vi "log analysis_gps.vi"() -> ()   [LabVIEW 2019] (continued)
\n\t\n15:46:26.6\tlog_raw\tgps_raw\t#INSPVAXA,USB3,0,50.5,FINESTEERING,2107,283604.650,02000000,471d,15824;INS_ALIGNMENT_COMPLETE,INS_RTKFIXED,37.37126199805,126.72219243143,7.9649,22.3000,0.0555,0.0695,0.0079,0.560896506,-1.435960650,267.028457385,0.4379,0.2961,0.5759,0.1131,0.0925,0.0784,0.0963,0.1009,5.1528,0f000001,0*81aa449e\n\tsystem status\tnormal 2 27.900000 0 0\trobot status\t120.229744\t125.611680\t7.964900\t0.560897\t-1.435961\t-177.028457\t-0.015000\t0.004000\n\t\n15:46:27.1\tlog_raw\tgps_raw\t\tsystem status\tnormal 2 27.900000 0 0\trobot status\t120.247613\t125.622386\t7.963000\t0.540052\t-1.322126\t-177.100128\t0.000000\t0.000000\n\t\n15:46:27.6\tlog_raw\tgps_raw\t\tsystem status\tnormal 2 27.900000 0 0\trobot status\t120.240000\t125.629099\t7.960700\t0.528374\t-1.345188\t-177.091097\t-0.003000\t0.005000\n\t\n15:46:28.1\tlog_raw\tgps_raw\t\tsystem status\tnormal 2 27.900000 0 0\trobot status\t120.240346\t125.635985\t7.958800\t0.528065\t-1.344161\t-177.088301\t0.000000\t0.000000\n\t\n15:46:28.6\tlog_raw\tgps_raw\t\tsystem status\tnormal 2 27.900000 0 0\trobot status\t120.241214\t125.638419\t7.957500\t0.527317\t-1.343603\t-177.097018\t0.000000\t0.000000\n\t\n15:46:29.1\tlog_raw\tgps_raw\t#INSPVAXA,USB3,0,45.0,FINESTEERING,2107,283607.150,02000000,471d,15824;INS_ALIGNMENT_COMPLETE,INS_RTKFIXED,37.37126226214,126.72219256337,7.9563,22.3000,0.0507,-0.0122,0.0067,0.527133772,-1.343948140,267.105174531,0.4402,0.2962,0.5756,0.1140,0.0925,0.0784,0.0963,0.1009,5.1518,0f000001,0*37532215\n\tsystem status\tnormal 2 27.900000 0 0\trobot status\t120.241431\t125.640990\t7.956300\t0.527134\t-1.343948\t-177.105175\t0.000000\t0.000000\n\t\n15:46:29.6\tlog_raw\tgps_raw\t#INSPVAXA,USB3,0,45.0,FINESTEERING,2107,283607.650,02000000,471d,15824;INS_ALIGNMENT_COMPLETE,INS_RTKFIXED,37.37126225847,126.72219257288,7.9545,22.3000,0.0487,-0.0117,0.0063,0.526769970,-1.341614130,267.120484585,0.4402,0.2962,0.5756,0.1140,0.0925,0.0784,0.0963,0.1009,5.1518,0f000001,0*097e3cbc\n\tsystem status\tnormal 2 27.900000 0 0\trobot status\t120.242273\t125.640582\t7.954500\t0.526770\t-1.341614\t-177.120485\t0.000000\t0.000000\n\t\n15:46:30.1\tlog_raw\tgps_raw\t\tsystem status\tnormal 2 27.900000 0 0\trobot status\t120.242654\t125.640475\t7.952800\t0.525450\t-1.341849\t-177.138025\t0.000000\t0.000000\n\t\n15:46:30.6\tlog_raw\tgps_raw\t\tsystem status\tnormal 2 27.900000 0 0\trobot status\t120.243154\t125.638122\t7.950900\t0.525220\t-1.343908\t-177.155087\t0.000000\t0.000000\n\t\n15:46:31.1\tlog_raw\tgps_raw\t\tsystem status\tnormal 2 27.900000 0 0\trobot status\t120.243352\t125.636540\t7.949400\t0.526035\t-1.344537\t-177.171645\t0.000000\t0.000000\n\t\n15:46:31.6\tlog_raw\tgps_raw\t\tsystem status\tnormal 2 27.900000 0 0\trobot status\t120.243773\t125.634214\t7.948000\t0.525760\t-1.343630\t-177.189591\t0.000000\t0.000000\n\t\n15:46:32.1\tlog_raw\tgps_raw\t\tsystem status\tnormal 2 27.900000 0 0\trobot status\t120.244034\t125.632347\t7.946800\t0.526232\t-1.341058\t-177.213820\t0.031000\t0.016000\n\t\n15:46:32.6\tlog_raw\tgps_raw\t\tsystem status\tnormal 2 27.800000 0 0\trobot status\t120.157560\t125.623590\t7.944400\t0.518356\t-1.205486\t-177.172033\t0.334000\t0.069000\n\t\n15:46:33.1\tlog_raw\tgps_raw\t\tsystem status\tnormal 2 27.900000 0 0\trobot status\t119.992825\t125.615194\t7.941000\t0.761003\t-1.235075\t-177.213040\t0.247000\t0.083000\n\t\n15:46:33.6\tlog_raw\tgps_raw\t\tsystem status\tnormal 2 27.800000 0 0\trobot status\t119.859694\t125.608416\t7.939500\t0.865415\t-0.962854\t-177.206885\t0.328000\t0.009000\n\t\n15:46:34.1\tlog_raw\tgps_raw\t\tsystem status\tnormal 2 27.900000 0 0\trobot status\t119.720756\t125.602946\t7.937700\t0.944420\t-0.675187\t-177.209566\t0.305000\t-0.006000\n\t\n15:46:34.6\tlog_raw\tgps_raw\t\tsystem status\tnormal 2 27.900000 0 0\trobot status\t119.607706\t125.601145\t7.935300\t1.235838\t-0.694517\t-176.982274\t0.053000\t0.017000\n\t\n15:46:35.2\tlog_raw\tgps_raw\t\tsystem status\tnormal 2 27.900000 0 0\trobot status\t119.498199\t125.596969\t7.933300\t1.155764\t-0.364011\t-177.058938\t0.315000\t0.047000\n\t\n15:46:35.7\tlog_raw\tgps_raw\t\tsystem status\tnormal 2 27.800000 0 0\trobot status\t119.370674\t125.593736\t7.932700\t1.037480\t-0.074198\t-176.883392\t0.323000\t0.000000\n\t\n15:46:36.2\tlog_raw\tgps_raw\t\tsystem status\tnormal 2 27.800000 0 0\trobot status\t119.227990\t125.592351\t7.933400\t1.079023\t0.069605\t-176.833003\t0.331000\t-0.050000\n\t\n15:46:36.7\tlog_raw\tgps_raw\t\tsystem status\tnormal 2 27.900000 0 0\trobot status\t119.087343\t125.592838\t7.934300\t1.129008\t0.093647\t-176.796316\t0.344000\t-0.082000\n\t\n15:46:37.2\tlog_raw\tgps_raw\t\tsystem status\tnormal 2 27.900000 0 0\trobot status\t118.945543\t125.594297\t7.935700\t1.235778\t0.057060\t-176.780369\t0.373000\t-0.127000\n\t\n15:46:37.7\tlog_raw\tgps_raw\t\tsystem status\tnormal 2 27.900000 0 0\trobot status\t118.803696\t125.594493\t7.937600\t1.216235\t-0.108384\t-176.748954\t0.357000\t-0.086000\n\t\n15:46:38.2\tlog_raw\tgps_raw\t\tsystem status\tnormal 2 27.800000 0 0\trobot status\t118.664225\t125.596035\t7.939400\t1.263594\t-0.402279\t-176.659906\t0.284000\t0.032000\n\t\n15:46:38.7\tlog_raw\tgps_raw\t\tsystem status\tnormal 2 27.900000 0 0\trobot status\t118.524850\t125.597283\t7.939600\t1.404144\t-0.659021\t-176.624250\t0.281000\t0.019000\n\t\n15:46:39.2\tlog_raw\tgps_raw\t\tsystem status\tnormal 2 27.900000 0 0\trobot status\t118.381157\t125.599793\t7.940000\t1.598406\t-0.888086\t-176.601260\t0.360000\t-0.098000\n\t\n15:46:39.7\tlog_raw\tgps_raw\t\tsystem status\tnormal 2 27.800000 0 0\trobot status\t118.277291\t125.603881\t7.941400\t1.566580\t-0.870870\t-176.521281\t0.316000\t0.024000\n\t\n15:46:40.2\tlog_raw\tgps_raw\t\tsystem status\tnormal 2 27.900000 0 0\trobot status\t118.128647\t125.607002\t7.942100\t1.627827\t-0.936186\t-176.519460\t0.217000\t0.054000\n\t\n15:46:40.7\tlog_raw\tgps_raw\t\tsystem status\tnormal 2 27.900000 0 0\trobot status\t117.982836\t125.609853\t7.941800\t1.720683\t-0.789013\t-176.481119\t0.260000\t0.048000\n\t\n15:46:41.2\tlog_raw\tgps_raw\t\tsystem status\tnormal 2 27.900000 0 0\trobot status\t117.844520\t125.613894\t7.942800\t1.697089\t-0.531895\t-176.383127\t0.285000\t0.052000\n\t\n15:46:41.7\tlog_raw\tgps_raw\t#INSPVAXA,USB3,0,49.5,FINESTEERING,2107,283619.700,02000000,471d,15824;INS_ALIGNMENT_COMPLETE,INS_RTKFIXED,37.37126206039,126.72216378783,7.9456,22.3000,0.0422,-0.2948,0.0158,1.718323220,-0.193748450,266.266037782,0.4350,0.2957,0.5763,0.1125,0.0925,0.0784,0.0965,0.1009,5.1330,0f000001,0*8635b490\n\tsystem status\tnormal 2 27.800000 0 0\trobot status\t117.692541\t125.618635\t7.945600\t1.718323\t-0.193748\t-176.266038\t0.383000\t-0.099000\n\t\n15:46:42.2\tlog_raw\tgps_raw\t\tsystem status\tnormal 2 27.800000 0 0\trobot status\t117.566611\t125.621702\t7.946700\t1.591710\t-0.089350\t-176.226869\t0.365000\t-0.094000\n\t\n15:46:42.7\tlog_raw\tgps_raw\t\tsystem status\tnormal 2 27.800000 0 0\trobot status\t117.417289\t125.623343\t7.946200\t1.490039\t-0.163044\t-176.175266\t0.376000\t-0.104000\n\t\n15:46:43.2\tlog_raw\tgps_raw\t\tsystem status\tnormal 2 27.800000 0 0\trobot status\t117.272242\t125.625795\t7.946400\t1.307058\t-0.220578\t-176.105754\t0.263000\t0.075000\n\t\n15:46:43.7\tlog_raw\tgps_raw\t\tsystem status\tnormal 2 27.800000 0 0\trobot status\t117.130621\t125.627578\t7.947200\t1.149741\t-0.274212\t-175.977532\t0.361000\t-0.089000\n\t\n15:46:44.2\tlog_raw\tgps_raw\t#INSPVAXA,USB3,0,47.5,FINESTEERING,2107,283622.200,02000000,471d,15824;INS_ALIGNMENT_COMPLETE,INS_RTKFIXED,37.37126217486,126.72215605148,7.9488,22.3000,0.0265,-0.2568,0.0016,0.953197769,-0.264991418,265.735651965,0.4362,0.2956,0.5763,0.1134,0.0927,0.0784,0.0965,0.1010,5.1347,0f000001,0*d1c7aea0\n\tsystem status\tnormal 2 27.800000 0 0\trobot status\t117.007267\t125.631349\t7.948800\t0.953198\t-0.264991\t-175.735652\t0.219000\t0.009000\n\t\n15:46:44.7\tlog_raw\tgps_raw\t\tsystem status\tnormal 2 27.800000 0 0\trobot status\t116.858071\t125.629441\t7.947800\t0.820028\t-0.582510\t-175.730144\t0.220000\t0.076000\n\t\n15:46:45.2\tlog_raw\tgps_raw\t#INSPVAXA,USB3,0,49.5,FINESTEERING,2107,283623.200,02000000,471d,15824;INS_ALIGNMENT_COMPLETE,INS_RTKFIXED,37.37126215352,126.72215258792,7.9480,22.3000,0.0351,-0.2613,0.0231,0.659350525,-0.553290360,265.516937653,0.4377,0.2954,0.5765,0.1123,0.0931,0.0784,0.0965,0.1010,5.1353,0f000001,0*f37e3ed0\n\tsystem status\tnormal 2 27.800000 0 0\trobot status\t116.700471\t125.628985\t7.948000\t0.659351\t-0.553290\t-175.516938\t0.236000\t0.095000\n\t\n15:46:45.7\tlog_raw\tgps_raw\t\tsystem status\tnormal 2 27.800000 0 0\trobot status\t116.570534\t125.627968\t7.947400\t0.491368\t-0.548221\t-175.479442\t0.356000\t-0.073000\n\t\n15:46:46.2\tlog_raw\tgps_raw\t\tsystem status\tnormal 2 27.800000 0 0\trobot status\t116.422797\t125.627372\t7.946500\t0.429298\t-0.761102\t-175.343158\t0.340000\t-0.050000\n\t\n15:46:46.7\tlog_raw\tgps_raw\t\tsystem status\tnormal 2 27.800000 0 0\trobot status\t116.278573\t125.625026\t7.945600\t0.327130\t-0.869350\t-175.264091\t0.333000\t-0.039000\n\t\n15:46:47.2\tlog_raw\tgps_raw\t#INSPVAXA,USB3,0,49.5,FINESTEERING,2107,283625.200,02000000,471d,15824;INS_ALIGNMENT_COMPLETE,INS_RTKFIXED,37.37126210638,126.72214606046,7.9447,22.3000,0.0217,-0.2754,0.0073,0.236515804,-0.792213520,265.180407825,0.4366,0.2950,0.5766,0.1123,0.0931,0.0784,0.0964,0.1010,5.1329,0f000001,0*acc95a4e\n\tsystem status\tnormal 2 27.800000 0 0\trobot status\t116.122279\t125.623761\t7.944700\t0.236516\t-0.792214\t-175.180408\t0.347000\t-0.074000\n\t\n15:46:47.7\tlog_raw\tgps_raw\t#INSPVAXA,USB3,0,49.5,FINESTEERING,2107,283625.700,02000000,471d,15824;INS_ALIGNMENT_COMPLETE,INS_RTKFIXED,37.37126208247,126.72214443464,7.9445,22.3000,0.0140,-0.2813,0.0048,0.046048670,-0.588797871,265.114785763,0.4366,0.2950,0.5766,0.1123,0.0931,0.0784,0.0964,0.1010,5.1329,0f000001,0*ce0a2a96\n\tsystem status\tnormal 2 27.800000 0 0\trobot status\t115.978267\t125.621109\t7.944500\t0.046049\t-0.588798\t-175.114786\t0.250000\t0.075000\n\t\n15:46:48.2\tlog_raw\tgps_raw\t#INSPVAXA,USB3,0,48.0,FINESTEERING,2107,283626.200,02000000,471d,15824;INS_ALIGNMENT_COMPLETE,INS_RTKFIXED,37.37126206372,126.72214280060,7.9445,22.3000,0.0212,-0.2855,0.0048,-0.004156486,-0.311026110,265.065225665,0.4366,0.2949,0.5766,0.1123,0.0931,0.0784,0.0963,0.1010,5.1300,0f000001,0*7442e942\n\tsystem status\tnormal 2 27.900000 0 0\trobot status\t115.833526\t125.619030\t7.944500\t-0.004156\t-0.311026\t-175.065226\t0.377000\t-0.106000\n\t\n15:46:48.7\tlog_raw\tgps_raw\t\tsystem status\tnormal 2 27.800000 0 0\trobot status\t115.708474\t125.615805\t7.943800\t-0.132371\t0.068230\t-174.996675\t0.252000\t0.082000\n\t\n15:46:49.2\tlog_raw\tgps_raw\t#INSPVAXA,USB3,0,48.5,FINESTEERING,2107,283627.200,02000000,471d,15824;INS_ALIGNMENT_COMPLETE,INS_RTKFIXED,37.37126201142,126.72213963218,7.9431,22.3000,0.0278,-0.2914,0.0131,-0.197757356,0.430555181,264.900646420,0.4366,0.2949,0.5768,0.1127,0.0931,0.0784,0.0962,0.1009,5.1266,0f000001,0*c875f714\n\tsystem status\tnormal 2 27.800000 0 0\trobot status\t115.552873\t125.613230\t7.943100\t-0.197757\t0.430555\t-174.900646\t0.372000\t-0.099000\n\t\n15:46:49.7\tlog_raw\tgps_raw\t\tsystem status\tnormal 2 27.800000 0 0\trobot status\t115.421996\t125.610470\t7.941400\t-0.273360\t0.391133\t-174.920780\t0.299000\t0.008000\n\t\n15:46:50.2\tlog_raw\tgps_raw\t\tsystem status\tnormal 2 27.900000 0 0\trobot status\t115.278884\t125.608053\t7.940600\t-0.346212\t0.271634\t-174.916641\t0.299000\t0.000000\n\t\n15:46:50.7\tlog_raw\tgps_raw\t#INSPVAXA,USB3,0,48.0,FINESTEERING,2107,283628.700,02000000,471d,15824;INS_ALIGNMENT_COMPLETE,INS_RTKFIXED,37.37126191178,126.72213473323,7.9380,22.3000,0.0177,-0.2797,-0.0032,-0.623534384,0.011887408,264.986854356,0.4375,0.2949,0.5768,0.1127,0.0930,0.0784,0.0962,0.1009,5.1221,0f000001,0*2b23c567\n\tsystem status\tnormal 2 27.900000 0 0\trobot status\t115.118932\t125.602177\t7.938000\t-0.623534\t0.011887\t-174.986854\t0.294000\t0.000000\n\t\n15:46:51.2\tlog_raw\tgps_raw\t#INSPVAXA,USB3,0,44.0,FINESTEERING,2107,283629.200,02000000,471d,15824;INS_ALIGNMENT_COMPLETE,INS_RTKFIXED,37.37126187751,126.72213308389,7.9364,22.3000,0.0207,-0.2899,-0.0036,-0.719101472,-0.426401600,265.021502859,0.4380,0.2949,0.5768,0.1123,0.0930,0.0784,0.0961,0.1009,5.1171,0f000001,0*92ebbc5f\n\tsystem status\tnormal 2 27.900000 0 0\trobot status\t114.972836\t125.598376\t7.936400\t-0.719101\t-0.426402\t-175.021503\t0.296000\t0.002000\n\t\n15:46:51.7\tlog_raw\tgps_raw\t#INSPVAXA,USB3,0,44.0,FINESTEERING,2107,283629.700,02000000,471d,15824;INS_ALIGNMENT_COMPLETE,INS_RTKFIXED,37.37126184367,126.72213142920,7.9356,22.3000,0.0231,-0.2981,-0.0100,-0.725013495,-0.732992105,265.121442983,0.4380,0.2949,0.5768,0.1123,0.0930,0.0784,0.0961,0.1009,5.1171,0f000001,0*6a5775b3\n\tsystem status\tnormal 2 27.900000 0 0\trobot status\t114.826266\t125.594622\t7.935600\t-0.725013\t-0.732992\t-175.121443\t0.302000\t0.000000\n\t\n15:46:52.2\tlog_raw\tgps_raw\t#INSPVAXA,USB3,0,47.0,FINESTEERING,2107,283630.200,02000000,471d,15824;INS_ALIGNMENT_COMPLETE,INS_RTKFIXED,37.37126181957,126.72212981940,7.9352,22.3000,0.0233,-0.2888,-0.0019,-0.675781239,-0.810566304,265.160131093,0.4376,0.2949,0.5768,0.1123,0.0928,0.0784,0.0961,0.1009,5.1128,0f000001,0*27ca04ea\n\tsystem status\tnormal 2 27.900000 0 0\trobot status\t114.683673\t125.591949\t7.935200\t-0.675781\t-0.810566\t-175.160131\t0.296000\t0.005000\n\t\n15:46:52.7\tlog_raw\tgps_raw\t#INSPVAXA,USB3,0,47.0,FINESTEERING,2107,283630.700,02000000,471d,15824;INS_ALIGNMENT_COMPLETE,INS_RTKFIXED,37.37126178591,126.72212819473,7.9347,22.3000,0.0150,-0.2861,-0.0012,-0.714770911,-0.869266848,265.221494891,0.4376,0.2949,0.5768,0.1123,0.0928,0.0784,0.0961,0.1009,5.1128,0f000001,0*aed2de40\n\tsystem status\tnormal 2 27.900000 0 0\trobot status\t114.539762\t125.588216\t7.934700\t-0.714771\t-0.869267\t-175.221495\t0.298000\t0.001000\n\t\n15:46:53.2\tlog_raw\tgps_raw\t#INSPVAXA,USB3,0,42.0,FINESTEERING,2107,283631.200,02000000,471d,15824;INS_ALIGNMENT_COMPLETE,INS_RTKFIXED,37.37126175832,126.72212651988,7.9323,22.3000,0.0193,-0.2829,-0.0000,-0.656726245,-0.814467356,265.316189024,0.4372,0.2950,0.5769,0.1123,0.0926,0.0784,0.0961,0.1009,5.1101,0f000001,0*d1b6c699\n\tsystem status\tnormal 2 27.900000 0 0\trobot status\t114.391407\t125.585156\t7.932300\t-0.656726\t-0.814467\t-175.316189\t0.295000\t-0.016000\n\t\n15:46:53.7\tlog_raw\tgps_raw\t#INSPVAXA,USB3,0,42.0,FINESTEERING,2107,283631.700,02000000,471d,15824;INS_ALIGNMENT_COMPLETE,INS_RTKFIXED,37.37126176860,126.72212533305,7.9296,22.3000,0.0361,-0.3378,-0.0103,-0.428138119,-0.668837581,265.144757660,0.4372,0.2950,0.5769,0.1123,0.0926,0.0784,0.0961,0.1009,5.1101,0f000001,0*53a99c66\n\tsystem status\tnormal 2 27.900000 0 0\trobot status\t114.286279\t125.586298\t7.929600\t-0.428138\t-0.668838\t-175.144758\t0.298000\t-0.003000\n\t\n15:46:54.2\tlog_raw\tgps_raw\t\tsystem status\tnormal 2 27.900000 0 0\trobot status\t114.123517\t125.583422\t7.925900\t-0.165245\t-0.957147\t-175.287983\t0.290000\t0.016000\n\t\n15:46:54.7\tlog_raw\tgps_raw\t#INSPVAXA,USB3,0,48.5,FINESTEERING,2107,283632.700,02000000,471d,15824;INS_ALIGNMENT_COMPLETE,INS_RTKFIXED,37.37126172516,126.72212196595,7.9217,22.3000,0.0261,-0.3154,-0.0017,-0.080275609,-1.010698207,265.307907457,0.4366,0.2951,0.5768,0.1127,0.0925,0.0784,0.0961,0.1008,5.1091,0f000001,0*c955826f\n\tsystem status\tnormal 2 27.900000 0 0\trobot status\t113.988027\t125.581481\t7.921700\t-0.080276\t-1.010698\t-175.307907\t0.298000\t-0.007000\n\t\n15:46:55.2\tlog_raw\tgps_raw\t#INSPVAXA,USB3,0,44.5,FINESTEERING,2107,283633.200,02000000,471d,15824;INS_ALIGNMENT_COMPLETE,INS_RTKFIXED,37.37126169079,126.72212014716,7.9199,22.3000,0.0199,-0.3002,0.0131,-0.062381377,-1.283391784,265.467989015,0.4356,0.2952,0.5768,0.1125,0.0925,0.0784,0.0961,0.1008,5.1096,0f000001,0*29ba6107\n\tsystem status\tnormal 2 27.900000 0 0\trobot status\t113.826921\t125.577668\t7.919900\t-0.062381\t-1.283392\t-175.467989\t0.302000\t-0.007000\n\t\n15:46:55.7\tlog_raw\tgps_raw\t#INSPVAXA,USB3,0,44.5,FINESTEERING,2107,283633.700,02000000,471d,15824;INS_ALIGNMENT_COMPLETE,INS_RTKFIXED,37.37126167129,126.72211861960,7.9201,22.3000,0.0266,-0.3162,-0.0026,-0.118708398,-1.041509272,265.462110158,0.4356,0.2952,0.5768,0.1125,0.0925,0.0784,0.0961,0.1008,5.1096,0f000001,0*f2130a3a\n\tsystem status\tnormal 2 27.900000 0 0\trobot status\t113.691613\t125.575506\t7.920100\t-0.118708\t-1.041509\t-175.462110\t0.303000\t0.002000\n\t\n15:46:56.2\tlog_raw\tgps_raw\t#INSPVAXA,USB3,0,50.5,FINESTEERING,2107,283634.200,02000000,471d,15824;INS_ALIGNMENT_COMPLETE,INS_RTKFIXED,37.37126166951,126.72211687193,7.9193,22.3000,0.0345,-0.2873,0.0162,0.231523125,-0.963780299,265.599746817,0.4352,0.2955,0.5769,0.1123,0.0929,0.0784,0.0961,0.1009,5.1105,0f000001,0*34468b3e\n\tsystem status\tnormal 2 27.900000 0 0\trobot status\t113.536807\t125.575311\t7.919300\t0.231523\t-0.963780\t-175.599747\t0.296000\t-0.010000\n\t\n15:46:56.7\tlog_raw\tgps_raw\t#INSPVAXA,USB3,0,50.5,FINESTEERING,2107,283634.700,02000000,471d,15824;INS_ALIGNMENT_COMPLETE,INS_RTKFIXED,37.37126165383,126.72211529605,7.9180,22.3000,0.0293,-0.3222,-0.0026,0.312038300,-0.626564523,265.688696868,0.4352,0.2955,0.5769,0.1123,0.0929,0.0784,0.0961,0.1009,5.1105,0f000001,0*7451a5d1\n\tsystem status\tnormal 2 27.900000 0 0\trobot status\t113.397218\t125.573572\t7.918000\t0.312038\t-0.626565\t-175.688697\t0.309000\t-0.004000\n\t\n15:46:57.2\tlog_raw\tgps_raw\t#INSPVAXA,USB3,0,48.5,FINESTEERING,2107,283635.200,02000000,471d,15824;INS_ALIGNMENT_COMPLETE,INS_RTKFIXED,37.37126163429,126.72211368866,7.9175,22.3000,0.0223,-0.3021,-0.0082,0.186097207,-0.250317479,265.804263291,0.4352,0.2960,0.5769,0.1124,0.0928,0.0784,0.0961,0.1009,5.1109,0f000001,0*57ac3a22\n\tsystem status\tnormal 2 27.900000 0 0\trobot status\t113.254838\t125.571406\t7.917500\t0.186097\t-0.250317\t-175.804263\t0.298000\t-0.006000\n\t\n15:46:57.7\tlog_raw\tgps_raw\t#INSPVAXA,USB3,0,48.5,FINESTEERING,2107,283635.700,02000000,471d,15824;INS_ALIGNMENT_COMPLETE,INS_RTKFIXED,37.37126159822,126.72211206599,7.9179,22.3000,0.0256,-0.3005,0.0044,-0.110995339,-0.087789516,265.935244450,0.4352,0.2960,0.5769,0.1124,0.0928,0.0784,0.0961,0.1009,5.1109,0f000001,0*fb1bd604\n\tsystem status\tnormal 2 27.900000 0 0\trobot status\t113.111105\t125.567404\t7.917900\t-0.110995\t-0.087790\t-175.935244\t0.296000\t-0.006000\n\t\n15:46:58.2\tlog_raw\tgps_raw\t\tsystem status\tnormal 2 27.900000 0 0\trobot status\t112.986609\t125.566337\t7.918000\t-0.168558\t-0.306352\t-176.034603\t0.281000\t0.003000\n\t\n15:46:58.7\tlog_raw\tgps_raw\t#INSPVAXA,USB3,0,43.0,FINESTEERING,2107,283636.700,02000000,471d,15824;INS_ALIGNMENT_COMPLETE,INS_RTKFIXED,37.37126158491,126.72210906167,7.9172,22.3000,0.0261,-0.3515,0.0074,-0.153804874,-0.423258614,266.149623913,0.4359,0.2963,0.5769,0.1124,0.0927,0.0784,0.0961,0.1009,5.1114,0f000001,0*20701ae8\n\tsystem status\tnormal 2 27.900000 0 0\trobot status\t112.844987\t125.565931\t7.917200\t-0.153805\t-0.423259\t-176.149624\t0.318000\t-0.009000\n\t\n15:46:59.2\tlog_raw\tgps_raw\t#INSPVAXA,USB3,0,48.5,FINESTEERING,2107,283637.200,02000000,471d,15824;INS_ALIGNMENT_COMPLETE,INS_RTKFIXED,37.37126157389,126.72210741579,7.9182,22.3000,0.0244,-0.2694,0.0184,-0.300056136,-0.600225307,266.307903185,0.4364,0.2964,0.5768,0.1122,0.0926,0.0784,0.0961,0.1009,5.1119,0f000001,0*6c5dc01c\n\tsystem status\tnormal 2 27.900000 0 0\trobot status\t112.699198\t125.564710\t7.918200\t-0.300056\t-0.600225\t-176.307903\t0.277000\t-0.009000\n\t\n15:46:59.7\tlog_raw\tgps_raw\t#INSPVAXA,USB3,0,48.5,FINESTEERING,2107,283637.700,02000000,471d,15824;INS_ALIGNMENT_COMPLETE,INS_RTKFIXED,37.37126156174,126.72210572455,7.9205,22.3000,0.0137,-0.2979,0.0107,-0.519565417,-0.746251495,266.511093088,0.4364,0.2964,0.5768,0.1122,0.0926,0.0784,0.0961,0.1009,5.1119,0f000001,0*d93f2085\n\tsystem status\tnormal 2 27.900000 0 0\trobot status\t112.549390\t125.563363\t7.920500\t-0.519565\t-0.746251\t-176.511093\t0.294000\t-0.009000\n\t\n15:47:00.2\tlog_raw\tgps_raw\t#INSPVAXA,USB3,0,51.0,FINESTEERING,2107,283638.200,02000000,471d,15824;INS_ALIGNMENT_COMPLETE,INS_RTKFIXED,37.37126155440,126.72210403454,7.9211,22.3000,0.0270,-0.3337,0.0126,-0.860556856,-0.781571793,266.718697356,0.4367,0.2965,0.5770,0.1123,0.0925,0.0784,0.0961,0.1009,5.1124,0f000001,0*3b4b6ae8\n\tsystem status\tnormal 2 27.900000 0 0\trobot status\t112.399692\t125.562551\t7.921100\t-0.860557\t-0.781572\t-176.718697\t0.302000\t-0.016000\n\t\n15:47:00.7\tlog_raw\tgps_raw\t#INSPVAXA,USB3,0,51.0,FINESTEERING,2107,283638.700,02000000,471d,15824;INS_ALIGNMENT_COMPLETE,INS_RTKFIXED,37.37126156669,126.72210242363,7.9200,22.3000,0.0334,-0.3133,0.0178,-0.896958447,-0.619411990,266.906112882,0.4367,0.2965,0.5770,0.1123,0.0925,0.0784,0.0961,0.1009,5.1124,0f000001,0*cef03a1f\n\tsystem status\tnormal 2 27.900000 0 0\trobot status\t112.257000\t125.563916\t7.920000\t-0.896958\t-0.619412\t-176.906113\t0.296000\t-0.004000\n\t\n15:47:01.2\tlog_raw\tgps_raw\t#INSPVAXA,USB3,0,50.0,FINESTEERING,2107,283639.200,02000000,471d,15824;INS_ALIGNMENT_COMPLETE,INS_RTKFIXED,37.37126157899,126.72210075579,7.9190,22.3000,0.0338,-0.2994,0.0184,-0.981388962,-0.616865309,267.067890648,0.4364,0.2961,0.5771,0.1123,0.0925,0.0784,0.0961,0.1009,5.1135,0f000001,0*21baf340\n\tsystem status\tnormal 2 27.900000 0 0\trobot status\t112.109266\t125.565284\t7.919000\t-0.981389\t-0.616865\t-177.067891\t0.292000\t0.000000\n\t\n15:47:01.7\tlog_raw\tgps_raw\t#INSPVAXA,USB3,0,50.0,FINESTEERING,2107,283639.700,02000000,471d,15824;INS_ALIGNMENT_COMPLETE,INS_RTKFIXED,37.37126158948,126.72209911436,7.9198,22.3000,0.0295,-0.3287,0.0146,-1.013704154,-0.682043166,267.265330343,0.4364,0.2961,0.5771,0.1123,0.0925,0.0784,0.0961,0.1009,5.1135,0f000001,0*ee73127b\n\tsystem status\tnormal 2 27.900000 0 0\trobot status\t111.963871\t125.566450\t7.919800\t-1.013704\t-0.682043\t-177.265330\t0.302000\t-0.009000\n\t\n15:47:02.2\tlog_raw\tgps_raw\t#INSPVAXA,USB3,0,49.5,FINESTEERING,2107,283640.200,02000000,471d,15824;INS_ALIGNMENT_COMPLETE,INS_RTKFIXED,37.37126161750,126.72209746371,7.9213,22.3000,0.0430,-0.3344,0.0134,-0.961284284,-0.929903840,267.457563863,0.4362,0.2958,0.5770,0.1123,0.0925,0.0784,0.0961,0.1009,5.1150,0f000001,0*e2e7a72b\n\tsystem status\tnormal 2 27.900000 0 0\trobot status\t111.817659\t125.569561\t7.921300\t-0.961284\t-0.929904\t-177.457564\t0.305000\t-0.007000\n\t\n15:47:02.7\tlog_raw\tgps_raw\t#INSPVAXA,USB3,0,49.5,FINESTEERING,2107,283640.700,02000000,471d,15824;INS_ALIGNMENT_COMPLETE,INS_RTKFIXED,37.37126164969,126.72209583664,7.9226,22.3000,0.0427,-0.3200,0.0053,-1.010366927,-1.135102181,267.635350069,0.4362,0.2958,0.5770,0.1123,0.0925,0.0784,0.0961,0.1009,5.1150,0f000001,0*6b674dca\n\tsystem status\tnormal 2 27.900000 0 0\trobot status\t111.673535\t125.573136\t7.922600\t-1.010367\t-1.135102\t-177.635350\t0.299000\t-0.002000\n\t\n15:47:03.2\tlog_raw\tgps_raw\t#DUALANTENNAHEADINGA,USB3,0,50.0,FINESTEERING,2107,283641.200,02000000,d426,15824;INSUFFICIENT_OBS,NONE,-1.000000000,0.000000000,0.000000000,0.0,0.000000000,0.000000000,\"631T\",11,4,4,3,04,00,20,02*472a6cda\n\tsystem status\tnormal 2 27.900000 0 0\trobot status\t111.525039\t125.579051\t7.923500\t-0.873522\t-1.303089\t-177.784444\t0.296000\t0.000000\n\t\n15:47:03.7\tlog_raw\tgps_raw\t#INSPVAXA,USB3,0,50.0,FINESTEERING,2107,283641.700,02000000,471d,15824;INS_ALIGNMENT_COMPLETE,INS_RTKFIXED,37.37126176584,126.72209246619,7.9228,22.3000,0.0335,-0.3477,0.0031,-0.698463635,-1.495934209,267.964863954,0.4360,0.2957,0.5769,0.1125,0.0925,0.0784,0.0961,0.1009,5.1165,0f000001,0*ca9d9e5e\n\tsystem status\tnormal 2 27.900000 0 0\trobot status\t111.374987\t125.586031\t7.922800\t-0.698464\t-1.495934\t-177.964864\t0.302000\t0.004000\n\t\n15:47:04.2\tlog_raw\tgps_raw\t#INSPVAXA,USB3,0,50.0,FINESTEERING,2107,283642.200,02000000,471d,15824;INS_ALIGNMENT_COMPLETE,INS_RTKFIXED,37.37126183344,126.72209071714,7.9215,22.3000,0.0370,-0.3263,0.0036,-0.535216936,-1.667310153,268.031771555,0.4354,0.2957,0.5768,0.1127,0.0926,0.0784,0.0961,0.1009,5.1177,0f000001,0*11bec665\n\tsystem status\tnormal 2 27.900000 0 0\trobot status\t111.220059\t125.593535\t7.921500\t-0.535217\t-1.667310\t-178.031772\t0.300000\t-0.003000\n\t\n15:47:04.7\tlog_raw\tgps_raw\t#DUALANTENNAHEADINGA,USB3,0,50.0,FINESTEERING,2107,283642.700,02000000,d426,15824;INSUFFICIENT_OBS,NONE,-1.000000000,0.000000000,0.000000000,0.0,0.000000000,0.000000000,\"631T\",12,4,4,3,04,00,20,03*f200c6d7\n\tsystem status\tnormal 2 27.900000 0 0\trobot status\t111.081969\t125.600643\t7.920400\t-0.422501\t-1.714756\t-178.135075\t0.296000\t0.006000\n\t\n15:47:05.2\tlog_raw\tgps_raw\t#DUALANTENNAHEADINGA,USB3,0,50.5,FINESTEERING,2107,283643.200,02000000,d426,15824;INSUFFICIENT_OBS,NONE,-1.000000000,0.000000000,0.000000000,0.0,0.000000000,0.000000000,\"631T\",14,4,4,3,04,00,20,02*f76a0e1e\n\tsystem status\tnormal 2 27.900000 0 0\trobot status\t110.939369\t125.607555\t7.918700\t-0.466356\t-1.548228\t-178.190993\t0.304000\t0.001000\n\t\n15:47:05.7\tlog_raw\tgps_raw\t#INSPVAXA,USB3,0,50.5,FINESTEERING,2107,283643.700,02000000,471d,15824;INS_ALIGNMENT_COMPLETE,INS_RTKFIXED,37.37126202513,126.72208597859,7.9183,22.3000,0.0299,-0.3163,0.0088,-0.418582783,-1.196326458,268.184941514,0.4349,0.2958,0.5767,0.1124,0.0926,0.0784,0.0961,0.1010,5.1181,0f000001,0*962e1d48\n\tsystem status\tnormal 2 27.900000 0 0\trobot status\t110.800326\t125.614816\t7.918300\t-0.418583\t-1.196326\t-178.184942\t0.297000\t0.006000\n\t\n15:47:06.2\tlog_raw\tgps_raw\t#INSPVAXA,USB3,0,50.0,FINESTEERING,2107,283644.200,02000000,471d,15824;INS_ALIGNMENT_COMPLETE,INS_RTKFIXED,37.37126209425,126.72208434200,7.9172,22.3000,0.0360,-0.2950,0.0056,-0.334802719,-0.884110622,268.233385323,0.4347,0.2959,0.5767,0.1122,0.0926,0.0784,0.0961,0.1010,5.1180,0f000001,0*78a9edf8\n\tsystem status\tnormal 2 27.900000 0 0\trobot status\t110.655359\t125.622489\t7.917200\t-0.334803\t-0.884111\t-178.233385\t0.299000\t-0.001000\n\t\n15:47:06.7\tlog_raw\tgps_raw\t#INSPVAXA,USB3,0,50.0,FINESTEERING,2107,283644.700,02000000,471d,15824;INS_ALIGNMENT_COMPLETE,INS_RTKFIXED,37.37126215178,126.72208275426,7.9159,22.3000,0.0303,-0.2952,0.0021,-0.296302250,-0.633495852,268.293666475,0.4347,0.2959,0.5767,0.1122,0.0926,0.0784,0.0961,0.1010,5.1180,0f000001,0*8db6baa1\n\tsystem status\tnormal 2 27.900000 0 0\trobot status\t110.514720\t125.628876\t7.915900\t-0.296302\t-0.633496\t-178.293666\t0.298000\t-0.001000\n\t\n15:47:07.2\tlog_raw\tgps_raw\t#INSPVAXA,USB3,0,46.0,FINESTEERING,2107,283645.200,02000000,471d,15824;INS_ALIGNMENT_COMPLETE,INS_RTKFIXED,37.37126220166,126.72208110110,7.9146,22.3000,0.0357,-0.3070,0.0007,-0.345507272,-0.608999756,268.311610368,0.4352,0.2960,0.5768,0.1123,0.0926,0.0784,0.0961,0.1011,5.1185,0f000001,0*f711e95a\n\tsystem status\tnormal 2 27.900000 0 0\trobot status\t110.368285\t125.634414\t7.914600\t-0.345507\t-0.609000\t-178.311610\t0.287000\t0.026000\n\t\n15:47:07.7\tlog_raw\tgps_raw\t#DUALANTENNAHEADINGA,USB3,0,46.0,FINESTEERING,2107,283645.700,02000000,d426,15824;INSUFFICIENT_OBS,NONE,-1.000000000,0.000000000,0.000000000,0.0,0.000000000,0.000000000,\"631T\",14,4,4,3,04,00,20,03*e6910734\n\tsystem status\tnormal 2 27.900000 0 0\trobot status\t110.227517\t125.638786\t7.914100\t-0.511260\t-0.771457\t-178.296151\t0.302000\t0.015000\n\t\n15:47:08.2\tlog_raw\tgps_raw\t#INSPVAXA,USB3,0,45.5,FINESTEERING,2107,283646.200,02000000,471d,15824;INS_ALIGNMENT_COMPLETE,INS_RTKFIXED,37.37126228996,126.72207792557,7.9145,22.3000,0.0424,-0.3064,0.0070,-0.583777876,-0.970443227,268.202528664,0.4357,0.2960,0.5768,0.1124,0.0925,0.0784,0.0961,0.1011,5.1194,0f000001,0*211ff137\n\tsystem status\tnormal 2 27.900000 0 0\trobot status\t110.087002\t125.644217\t7.914500\t-0.583778\t-0.970443\t-178.202529\t0.286000\t0.027000\n\t\n15:47:08.7\tlog_raw\tgps_raw\t#INSPVAXA,USB3,0,45.5,FINESTEERING,2107,283646.700,02000000,471d,15824;INS_ALIGNMENT_COMPLETE,INS_RTKFIXED,37.37126233833,126.72207631349,7.9144,22.3000,0.0451,-0.2992,0.0137,-0.600671632,-1.104685881,268.101292386,0.4357,0.2960,0.5768,0.1124,0.0925,0.0784,0.0961,0.1011,5.1194,0f000001,0*24418ec0\n\tsystem status\tnormal 2 27.900000 0 0\trobot status\t109.944207\t125.649587\t7.914400\t-0.600672\t-1.104686\t-178.101292\t0.253000\t0.080000\n\t\n15:47:09.2\tlog_raw\tgps_raw\t#DUALANTENNAHEADINGA,USB3,0,48.5,FINESTEERING,2107,283647.200,02000000,d426,15824;INSUFFICIENT_OBS,NONE,-1.000000000,0.000000000,0.000000000,0.0,0.000000000,0.000000000,\"631T\",13,4,4,3,04,00,20,03*e3593a63\n\tsystem status\tnormal 2 27.800000 0 0\trobot status\t109.798996\t125.654285\t7.915100\t-0.711305\t-1.244972\t-178.007017\t0.294000\t0.028000\n\t\n15:47:09.7\tlog_raw\tgps_raw\t#INSPVAXA,USB3,0,48.5,FINESTEERING,2107,283647.700,02000000,471d,15824;INS_ALIGNMENT_COMPLETE,INS_RTKFIXED,37.37126242655,126.72207309668,7.9156,22.3000,0.0394,-0.3060,0.0118,-0.639679760,-1.236455959,267.822984990,0.4363,0.2960,0.5769,0.1123,0.0925,0.0784,0.0961,0.1011,5.1206,0f000001,0*6bb51677\n\tsystem status\tnormal 2 27.800000 0 0\trobot status\t109.659267\t125.659382\t7.915600\t-0.639680\t-1.236456\t-177.822985\t0.313000\t-0.004000\n\t\n15:47:10.2\tlog_raw\tgps_raw\t#INSPVAXA,USB3,0,48.0,FINESTEERING,2107,283648.200,02008000,471d,15824;INS_ALIGNMENT_COMPLETE,INS_RTKFIXED,37.37126246801,126.72207154325,7.9155,22.3000,0.0354,-0.2935,0.0108,-0.510675062,-1.137543161,267.571098751,0.4364,0.2959,0.5770,0.1124,0.0925,0.0784,0.0961,0.1011,5.1221,0f000001,0*c4dadb2f\n\tsystem status\tnormal 2 27.800000 0 0\trobot status\t109.521667\t125.663985\t7.915500\t-0.510675\t-1.137543\t-177.571099\t0.406000\t-0.159000\n\t\n15:47:10.7\tlog_raw\tgps_raw\t#INSPVAXA,USB3,0,48.0,FINESTEERING,2107,283648.700,02008000,471d,15824;INS_ALIGNMENT_COMPLETE,INS_RTKFIXED,37.37126248707,126.72206994787,7.9152,22.3000,0.0198,-0.2907,0.0205,-0.532213630,-1.121566976,267.351964744,0.4364,0.2959,0.5770,0.1124,0.0925,0.0784,0.0961,0.1011,5.1221,0f000001,0*5feed5da\n\tsystem status\tnormal 2 27.800000 0 0\trobot status\t109.380351\t125.666103\t7.915200\t-0.532214\t-1.121567\t-177.351965\t0.257000\t0.071000\n\t\n15:47:11.2\tlog_raw\tgps_raw\t#INSPVAXA,USB3,0,50.5,FINESTEERING,2107,283649.200,02008000,471d,15824;INS_ALIGNMENT_COMPLETE,INS_RTKFIXED,37.37126248971,126.72206839810,7.9149,22.3000,0.0089,-0.2933,0.0096,-0.659725734,-0.970229399,267.160180872,0.4369,0.2958,0.5772,0.1125,0.0925,0.0784,0.0961,0.1011,5.1235,0f000001,0*081a7c85\n\tsystem status\tnormal 2 27.800000 0 0\trobot status\t109.243075\t125.666397\t7.914900\t-0.659726\t-0.970229\t-177.160181\t0.269000\t0.067000\n\t\n15:47:11.7\tlog_raw\tgps_raw\t#INSPVAXA,USB3,0,50.5,FINESTEERING,2107,283649.700,02008000,471d,15824;INS_ALIGNMENT_COMPLETE,INS_RTKFIXED,37.37126248182,126.72206686817,7.9130,22.3000,0.0195,-0.2818,0.0147,-0.676677557,-0.877493738,266.924781860,0.4369,0.2958,0.5772,0.1125,0.0925,0.0784,0.0961,0.1011,5.1235,0f000001,0*7b64dc48\n\tsystem status\tnormal 2 27.800000 0 0\trobot status\t109.107556\t125.665523\t7.913000\t-0.676678\t-0.877494\t-176.924782\t0.304000\t0.005000\n\t\n15:47:12.2\tlog_raw\tgps_raw\t#INSPVAXA,USB3,0,51.0,FINESTEERING,2107,283650.200,02008000,471d,15824;INS_ALIGNMENT_COMPLETE,INS_RTKFIXED,37.37126249199,126.72206547845,7.9115,22.3000,0.0164,-0.3260,0.0139,-0.484645802,-0.829453687,266.635151565,0.4374,0.2957,0.5772,0.1135,0.0925,0.0784,0.0961,0.1011,5.1243,0f000001,0*b0320f40\n\tsystem status\tnormal 2 27.800000 0 0\trobot status\t108.984457\t125.666654\t7.911500\t-0.484646\t-0.829454\t-176.635152\t0.250000\t0.091000\n\t\n15:47:12.7\tlog_raw\tgps_raw\t#INSPVAXA,USB3,0,51.0,FINESTEERING,2107,283650.700,02008000,471d,15824;INS_ALIGNMENT_COMPLETE,INS_RTKFIXED,37.37126248591,126.72206385137,7.9107,22.3000,0.0102,-0.2983,0.0161,-0.427862387,-0.984462668,266.224829667,0.4374,0.2957,0.5772,0.1135,0.0925,0.0784,0.0961,0.1011,5.1243,0f000001,0*ccab10f5\n\tsystem status\tnormal 2 27.800000 0 0\trobot status\t108.840333\t125.665981\t7.910700\t-0.427862\t-0.984463\t-176.224830\t0.318000\t-0.010000\n\t\n15:47:13.2\tlog_raw\tgps_raw\t#INSPVAXA,USB3,0,46.5,FINESTEERING,2107,283651.200,02008000,471d,15824;INS_ALIGNMENT_COMPLETE,INS_RTKFIXED,37.37126247297,126.72206225341,7.9105,22.3000,-0.0025,-0.2931,0.0133,-0.399154165,-1.231884130,265.791711510,0.4388,0.2958,0.5773,0.1125,0.0926,0.0784,0.0961,0.1010,5.1233,0f000001,0*02f453ca\n\tsystem status\tnormal 2 27.700000 0 0\trobot status\t108.698788\t125.664547\t7.910500\t-0.399154\t-1.231884\t-175.791712\t0.370000\t-0.093000\n\t\n15:47:13.7\tlog_raw\tgps_raw\t#DUALANTENNAHEADINGA,USB3,0,46.5,FINESTEERING,2107,283651.700,02008000,d426,15824;INSUFFICIENT_OBS,NONE,-1.000000000,0.000000000,0.000000000,0.0,0.000000000,0.000000000,\"631T\",12,4,4,3,04,00,20,02*dcd0f98d\n\tsystem status\tnormal 2 27.800000 0 0\trobot status\t108.558481\t125.661874\t7.910200\t-0.466368\t-1.539529\t-175.264272\t0.302000\t0.009000\n\t\n15:47:14.2\tlog_raw\tgps_raw\t#DUALANTENNAHEADINGA,USB3,0,52.0,FINESTEERING,2107,283652.200,02000000,d426,15824;INSUFFICIENT_OBS,NONE,-1.000000000,0.000000000,0.000000000,0.0,0.000000000,0.000000000,\"631T\",13,4,4,3,04,00,20,03*c51a48ea\n\tsystem status\tnormal 2 27.700000 0 0\trobot status\t108.415346\t125.659730\t7.909700\t-0.308960\t-1.712657\t-174.851669\t0.259000\t0.064000\n\t\n15:47:14.7\tlog_raw\tgps_raw\t#INSPVAXA,USB3,0,52.0,FINESTEERING,2107,283652.700,02000000,471d,15824;INS_ALIGNMENT_COMPLETE,INS_RTKFIXED,37.37126238850,126.72205745647,7.9080,22.3000,0.0144,-0.2874,0.0010,-0.261960509,-1.758395569,264.562436767,0.4386,0.2958,0.5773,0.1122,0.0925,0.0784,0.0961,0.1009,5.1223,0f000001,0*48b75177\n\tsystem status\tnormal 2 27.800000 0 0\trobot status\t108.273883\t125.655177\t7.908000\t-0.261961\t-1.758396\t-174.562437\t0.243000\t0.113000\n\t\n15:47:15.2\tlog_raw\tgps_raw\t#DUALANTENNAHEADINGA,USB3,0,49.5,FINESTEERING,2107,283653.200,02000000,d426,15824;INSUFFICIENT_OBS,NONE,-1.000000000,0.000000000,0.000000000,0.0,0.000000000,0.000000000,\"631T\",12,4,4,3,04,00,20,02*b48bfb58\n\tsystem status\tnormal 2 27.800000 0 0\trobot status\t108.136477\t125.650270\t7.905900\t-0.264942\t-1.676339\t-174.267820\t0.286000\t0.022000\n\t\n15:47:15.7\tlog_raw\tgps_raw\t#DUALANTENNAHEADINGA,USB3,0,49.5,FINESTEERING,2107,283653.700,02000000,d426,15824;INSUFFICIENT_OBS,NONE,-1.000000000,0.000000000,0.000000000,0.0,0.000000000,0.000000000,\"631T\",11,4,4,3,04,00,20,03*b7c95c3e\n\tsystem status\tnormal 2 27.800000 0 0\trobot status\t107.997731\t125.643866\t7.903800\t-0.357288\t-1.386075\t-174.083039\t0.254000\t0.063000\n\t\n15:47:16.2\tlog_raw\tgps_raw\t#DUALANTENNAHEADINGA,USB3,0,45.0,FINESTEERING,2107,283654.200,02000000,d426,15824;INSUFFICIENT_OBS,NONE,-1.000000000,0.000000000,0.000000000,0.0,0.000000000,0.000000000,\"631T\",11,4,4,3,04,00,20,03*317f5696\n\tsystem status\tnormal 2 27.800000 0 0\trobot status\t107.856218\t125.638907\t7.903000\t-0.193840\t-1.249928\t-173.972465\t0.295000\t0.006000\n\t\n15:47:16.7\tlog_raw\tgps_raw\t#DUALANTENNAHEADINGA,USB3,0,45.0,FINESTEERING,2107,283654.700,02000000,d426,15824;INSUFFICIENT_OBS,NONE,-1.000000000,0.000000000,0.000000000,0.0,0.000000000,0.000000000,\"631T\",12,4,4,3,04,00,20,03*453ac166\n\tsystem status\tnormal 2 27.800000 0 0\trobot status\t107.718981\t125.633996\t7.902900\t-0.104724\t-1.042235\t-173.990984\t0.367000\t-0.110000\n\t\n15:47:17.2\tlog_raw\tgps_raw\t#DUALANTENNAHEADINGA,USB3,0,47.5,FINESTEERING,2107,283655.200,02000000,d426,15824;INSUFFICIENT_OBS,NONE,-1.000000000,0.000000000,0.000000000,0.0,0.000000000,0.000000000,\"631T\",13,4,4,3,04,00,20,02*c2e72fac\n\tsystem status\tnormal 2 27.900000 0 0\trobot status\t107.581424\t125.629159\t7.902200\t-0.095623\t-0.778741\t-174.113632\t0.298000\t-0.023000\n\t\n15:47:17.7\tlog_raw\tgps_raw\t#DUALANTENNAHEADINGA,USB3,0,47.5,FINESTEERING,2107,283655.700,02000000,d426,15824;INSUFFICIENT_OBS,NONE,-1.000000000,0.000000000,0.000000000,0.0,0.000000000,0.000000000,\"631T\",11,4,4,3,04,00,20,03*16470892\n\tsystem status\tnormal 2 27.900000 0 0\trobot status\t107.440627\t125.622878\t7.900800\t-0.280891\t-0.708713\t-174.269259\t0.292000\t-0.007000\n\t\n15:47:18.2\tlog_raw\tgps_raw\t#DUALANTENNAHEADINGA,USB3,0,50.0,FINESTEERING,2107,283656.200,02000000,d426,15824;INSUFFICIENT_OBS,NONE,-1.000000000,0.000000000,0.000000000,0.0,0.000000000,0.000000000,\"631T\",11,4,4,3,04,00,20,02*6231c6e0\n\tsystem status\tnormal 2 27.900000 0 0\trobot status\t107.296655\t125.617070\t7.898700\t-0.492777\t-0.982858\t-174.397272\t0.296000\t-0.015000\n\t\n15:47:18.7\tlog_raw\tgps_raw\t#DUALANTENNAHEADINGA,USB3,0,50.0,FINESTEERING,2107,283656.700,02000000,d426,15824;INSUFFICIENT_OBS,NONE,-1.000000000,0.000000000,0.000000000,0.0,0.000000000,0.000000000,\"631T\",13,4,4,3,04,00,20,03*b691e1de\n\tsystem status\tnormal 2 27.900000 0 0\trobot status\t107.153389\t125.612301\t7.896600\t-0.613828\t-1.318461\t-174.520004\t0.298000\t-0.016000\n\t\n15:47:19.2\tlog_raw\tgps_raw\t#DUALANTENNAHEADINGA,USB3,0,48.0,FINESTEERING,2107,283657.200,02000000,d426,15824;INSUFFICIENT_OBS,NONE,-1.000000000,0.000000000,0.000000000,0.0,0.000000000,0.000000000,\"631T\",13,4,4,3,04,00,20,02*3e465e4d\n\tsystem status\tnormal 2 27.900000 0 0\trobot status\t107.015505\t125.610946\t7.894900\t-0.499571\t-1.452141\t-174.595468\t0.301000\t0.001000\n\t\n15:47:19.7\tlog_raw\tgps_raw\t#DUALANTENNAHEADINGA,USB3,0,48.0,FINESTEERING,2107,283657.700,02000000,d426,15824;INSUFFICIENT_OBS,NONE,-1.000000000,0.000000000,0.000000000,0.0,0.000000000,0.000000000,\"631T\",13,4,4,3,04,00,20,02*e9554f14\n\tsystem status\tnormal 2 27.900000 0 0\trobot status\t106.867329\t125.609513\t7.893600\t-0.474094\t-1.702577\t-174.750871\t0.300000\t0.008000\n\t\n15:47:20.2\tlog_raw\tgps_raw\t#INSPVAXA,USB3,0,51.0,FINESTEERING,2107,283658.200,02000000,471d,15824;INS_ALIGNMENT_COMPLETE,INS_RTKFIXED,37.37126197205,126.72203987070,7.8924,22.3000,0.0140,-0.2985,0.0088,-0.407757942,-1.836378522,264.980716512,0.4370,0.2959,0.5779,0.1123,0.0925,0.0785,0.0961,0.1008,5.1265,0f000001,0*c213c735\n\tsystem status\tnormal 2 27.900000 0 0\trobot status\t106.716164\t125.608978\t7.892400\t-0.407758\t-1.836379\t-174.980717\t0.301000\t0.000000\n\t\n15:47:20.7\tlog_raw\tgps_raw\t#DUALANTENNAHEADINGA,USB3,0,51.0,FINESTEERING,2107,283658.700,02000000,d426,15824;INSUFFICIENT_OBS,NONE,-1.000000000,0.000000000,0.000000000,0.0,0.000000000,0.000000000,\"631T\",14,4,4,3,04,00,20,02*806fba7a\n\tsystem status\tnormal 2 27.900000 0 0\trobot status\t106.573786\t125.609186\t7.890300\t-0.468031\t-1.661508\t-175.117193\t0.294000\t0.002000\n\t\n15:47:21.2\tlog_raw\tgps_raw\t#DUALANTENNAHEADINGA,USB3,0,45.5,FINESTEERING,2107,283659.200,02000000,d426,15824;INSUFFICIENT_OBS,NONE,-1.000000000,0.000000000,0.000000000,0.0,0.000000000,0.000000000,\"631T\",13,4,4,3,04,00,20,02*be5dbd8b\n\tsystem status\tnormal 2 27.900000 0 0\trobot status\t106.421661\t125.608502\t7.887500\t-0.499703\t-1.661370\t-175.263305\t0.310000\t-0.006000\n\t\n15:47:21.7\tlog_raw\tgps_raw\t#INSPVAXA,USB3,0,45.5,FINESTEERING,2107,283659.700,02000000,471d,15824;INS_ALIGNMENT_COMPLETE,INS_RTKFIXED,37.37126196302,126.72203492233,7.8846,22.3000,0.0219,-0.3038,0.0154,-0.352814130,-1.840091471,265.280226018,0.4363,0.2959,0.5779,0.1123,0.0925,0.0785,0.0961,0.1008,5.1280,0f000001,0*f5025ff3\n\tsystem status\tnormal 2 27.900000 0 0\trobot status\t106.277846\t125.607981\t7.884600\t-0.352814\t-1.840091\t-175.280226\t0.367000\t-0.092000\n\t\n15:47:22.2\tlog_raw\tgps_raw\t#DUALANTENNAHEADINGA,USB3,0,48.5,FINESTEERING,2107,283660.200,02000000,d426,15824;INSUFFICIENT_OBS,NONE,-1.000000000,0.000000000,0.000000000,0.0,0.000000000,0.000000000,\"631T\",14,4,4,3,04,00,20,02*21adfb59\n\tsystem status\tnormal 2 27.800000 0 0\trobot status\t106.135759\t125.606764\t7.883100\t-0.295459\t-1.820768\t-175.222439\t0.349000\t-0.082000\n\t\n15:47:22.7\tlog_raw\tgps_raw\t#DUALANTENNAHEADINGA,USB3,0,48.5,FINESTEERING,2107,283660.700,02000000,d426,15824;INSUFFICIENT_OBS,NONE,-1.000000000,0.000000000,0.000000000,0.0,0.000000000,0.000000000,\"631T\",15,4,4,3,04,00,20,03*565b5ace\n\tsystem status\tnormal 2 27.800000 0 0\trobot status\t105.990738\t125.602599\t7.883200\t-0.407735
